vi "Temperature Limit.vi"(3 "상위 리미트":dbl=80.0 format="%.2f", 4 "델터 t(ms)":u32=400 min=50 max=2000 step=50, 5 "수집할 포인트":i32=75 min=20 max=500) -> ()   [LabVIEW 2018]
doc: "이 VI는 온도 수집을 시뮬레이션하며, 온도를 그래프로 나타내며, 온도가 리미트보다 높은 경우, 사용자에게 이를 통지합니다.\n\n이 VI는 LabVIEW Basics II의 연습문제이며 프로퍼티 노드를 배우는데 사용됩니다."
panel:
  out "리미트 초과":bool
  in  "강제 종료":bool
  out "온도":cluster{"Temperature":dbl, "High Limit":dbl}(graph)
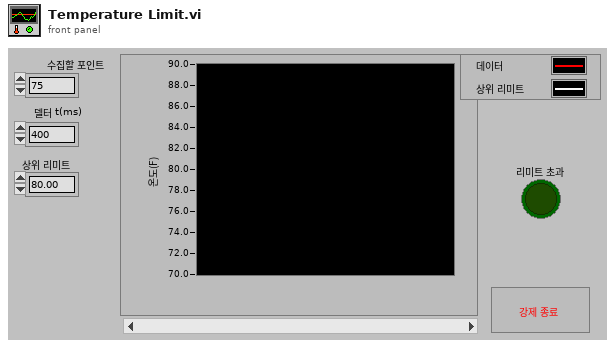
[diagram p1: front panel]
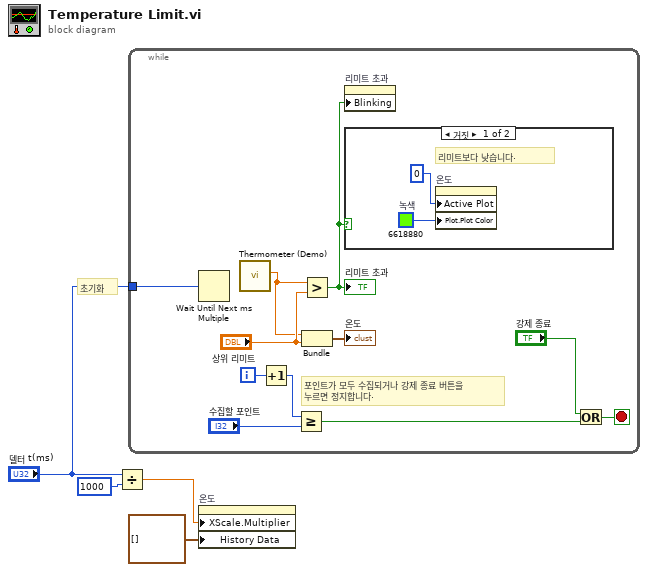
[diagram p0: block diagram]
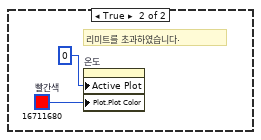
[diagram p2: hidden frame]
diagram:
  # "초기화"
  n1 = Divide(x="델터 t(ms)", y=1000) -> (x/y=w2:dbl)
  n2 = while {
    tunnel: "델터 t(ms)" -> [w7]
    i -> [w14]
    stop <- w8 stop-if-true
    # "포인트가 모두 수집되거나 강제 종료 버튼을 누르면 정지합니다."
    n3 = Wait Until Next ms Multiple(millisecond multiple=w7) -> ()  [unwired: 1 out]
    n4 = call "Thermometer (Demo).vi"() -> ("온도"=w5:dbl)  [unwired: 9 in, 1 out]
    n5 = Increment(x=w14) -> (x+1=w12:i32)
    n6 = Greater Or Equal?(x=w12, y="수집할 포인트") -> (x >= y?=w10:bool)
    n7 = Greater?(x=w5, y="상위 리미트") -> (0:w6:bool)
    "리미트 초과" <- w6
    n8 = Bundle("온도"=w5, "상위 리미트"="상위 리미트") -> (→"온도":cluster{"온도":dbl, "상위 리미트":dbl})  [unwired: 1 in]
    n9 = property on="리미트 초과" class="Bool (엄격한)"("Blinking"=w6) -> ()  [unwired: 2 in, 2 out]
    n10 = case shown="거짓" w6 {
      frame False {
        w16 = u32 6618880  # 녹색
        # "리미트보다 낮습니다."
        n11 = property on="온도" class="WFChart (엄격한)"("Active Plot"=0, "Plot.Plot Color"=w16) -> ()  [unwired: 2 in, 2 out]
      }
      frame True {
        w18 = u32 16711680  # 빨간색
        # "리미트를 초과하였습니다."
        n12 = property on="온도" class="WFChart (엄격한)"("Active Plot"=0, "Plot.Plot Color"=w18) -> ()  [unwired: 2 in, 2 out]
      }
    }
    n13 = Or(x="강제 종료", y=w10) -> (x .or. y?=w8:bool)
  }
  n14 = property on="온도" class="WFChart (엄격한)"("XScale.Multiplier"=w2, "History Data"=cluster{"Temperature":dbl, "High Limit":dbl}[] [] ("히스토리 데이터")) -> ()  [unwired: 2 in, 2 out]
